vi "Calibrate Polarizer.vi"(8 "error in (no error)":errorcluster, 11 "Application in":refnum<class "Application.lvclass">) -> (0 "error out":errorcluster, 3 "Application out":refnum<class "Application.lvclass">)   [LabVIEW 2023, in "Application.lvlib" / "Application.lvclass"]
uses:
  Application.lvclass
  Application.lvclass/Application.ctl
  Hardware/Thorlabs Polarizer Messages/Calibrate Polarizer Msg/Calibrate Polarizer Msg.lvclass
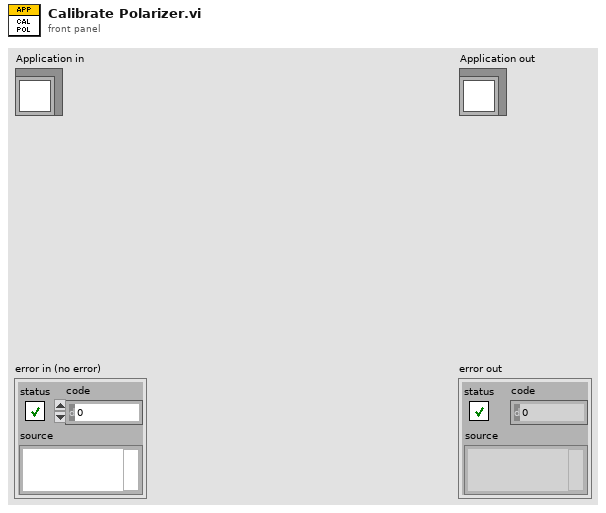
[diagram p1: front panel]
types:
  T1 = enum16{"Disable", "Laser Quantum", "Coherent OBIS", "PRM1-Z8", "Coherent HOPS"}
  T2 = typedef "Laser Configuration.ctl" = cluster{"Serial Port":refnum<visa-resource-name>, "Laser Type":enum16{"Disable", "Laser Quantum", "Coherent OBIS", "PRM1-Z8", "Coherent HOPS"}, "Polarizer Amplitude":dbl, "Polarizer Theta Zero":dbl, "Wavelength":u16}
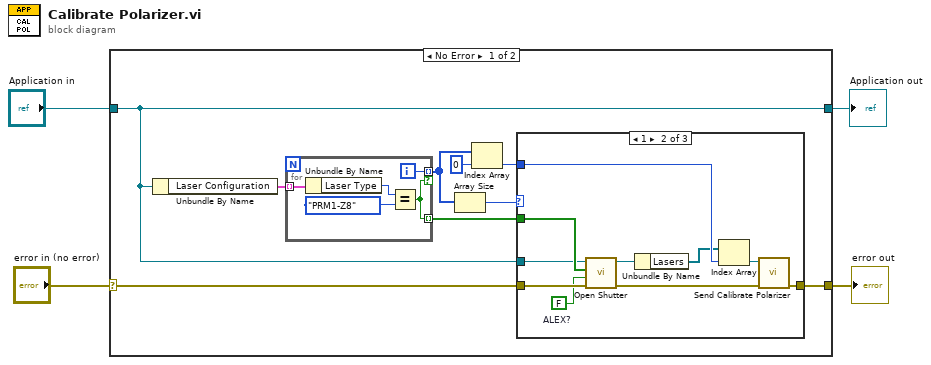
[diagram p0: block diagram]
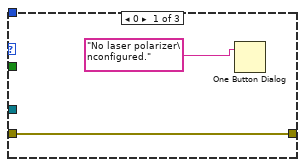
[diagram p2: hidden frame]
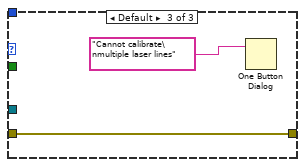
[diagram p3: hidden frame]
diagram:
  n1 = case shown="No Error" "error in (no error)" {
    selector: "error in (no error)" -> [w5 w33]
    tunnel: [w10 w33] -> w3
    tunnel: [w6 w32] -> w1
    tunnel: "Application in" -> [w6 w32]
    frame No Error {
      n2 = Unbundle By Name(w6) -> ("Laser Configuration"=w13:T2[])
      n3 = for {
        tunnel: w13 -> [w18] mode=indexing
        tunnel: [w15] -> w11 mode=indexing if=w14
        tunnel: [w14] -> w7 mode=indexing
        i -> [w15]
        n4 = Unbundle By Name(w18) -> ("Laser Type"=w17:T1)
        n5 = Equal?(x=w17, y=T1."PRM1-Z8") -> (x = y?=w14:bool)
      }
      n6 = Array Size(array=w11) -> (size(s)=w12:i32)
      n7 = Index Array(array=w11, index=0) -> (element=w8:i32)
      n8 = case shown="1" w12 {
        tunnel: [w19 w29 w30] -> w10
        tunnel: w8 -> [_ w27 _]
        tunnel: w5 -> [w19 w26 w30]
        tunnel: w6 -> [_ w22 _]
        tunnel: w7 -> [_ w23 _]
        frame 0 {
          n9 = One Button Dialog(message="No laser polarizer\nconfigured.") -> ()  [unwired: 1 in, 1 out]
        }
        frame 1 {
          w24 = FALSE  # ALEX?
          n10 = call-dynamic "Open Shutter.vi"("ALEX?"=w24, "Array"=w23, "Application in"=w22) -> ("Application out"=w21:refnum<class "Application.lvclass">)  [unwired: 7 in, 1 out]
          n11 = Unbundle By Name(w21) -> ("Lasers"=w25:refnum<class "Message Enqueuer.lvclass">[])
          n12 = Index Array(array=w25, index=w27) -> (element=w28:refnum<class "Message Enqueuer.lvclass">)
          n13 = call "Send Calibrate Polarizer.vi"("error in (no error)"=w26, "Message Enqueuer"=w28) -> ("error out"=w29:errorcluster)  [unwired: 8 in, 1 out]
        }
        frame Default {
          n14 = One Button Dialog(message="Cannot calibrate\nmultiple laser lines") -> ()  [unwired: 1 in, 1 out]
        }
      }
    }
    frame Error {
    }
  }
  "error out" <- w3
  "Application out" <- w1
